vi "Process.CreateRefs.vi"(7 "Default IDs":u32[](array[numeric]), 8 "error in (no error)":errorcluster, 10 "Port Settings":T1, 11 "Name":string) -> (0 "error out":errorcluster, 2 "FilterDVR.Ref":refnum<data-value>, 3 "Initial Settings":T5)   [LabVIEW 2025, in "xnet_can_bus_monitor_api_server_do.lvlib"]
uses:
  Types/XNET.InitialSettings.ctl
  xnet_can_bus_monitor_api_server/RPC Messages/ni_xnet_can_bm_api_ConnectSettings.ctl
  xnet_can_bus_monitor_api_server/RPC Messages/ni_xnet_can_bm_api_CanMode.ctl
  xnet_can_bus_monitor_api_server/RPC Messages/ni_xnet_can_bm_api_Termination.ctl
  xnet_can_bus_monitor_api_server/RPC Messages/ni_xnet_can_bm_api_FdIsoMode.ctl
  xnet_can_bus_monitor_api_server/RPC Messages/ni_xnet_can_bm_api_FilterInfo.ctl
  xnet_can_bus_monitor_api_server/RPC Messages/ni_xnet_can_bm_api_DirectionFilter.ctl
  xnet_can_bus_monitor_api_server/RPC Messages/ni_xnet_can_bm_api_FrameFilter.ctl
  xnet_can_bus_monitor_api_server_do.lvlib
  xnet_can_bus_monitor_api_server/xnet_can_bus_monitor_api_server.lvlib
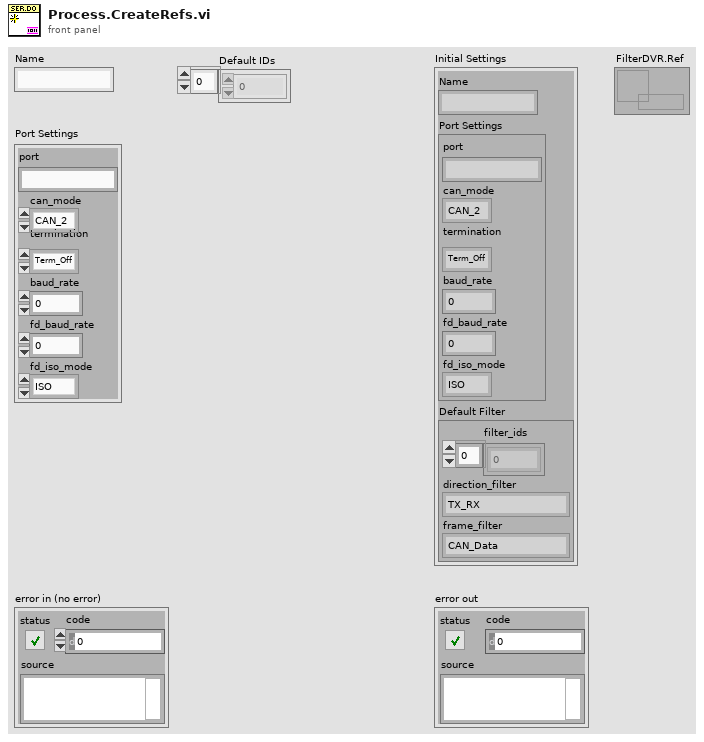
[diagram p1: front panel]
types:
  T1 = typedef "xnet_can_bus_monitor_api_server.lvlib/ni_xnet_can_bm_api_ConnectSettings.ctl" = cluster{"port":string, "can_mode":T2, "termination":T3, "baud_rate":u64, "fd_baud_rate":u64, "fd_iso_mode":T4}
  T2 = typedef "xnet_can_bus_monitor_api_server.lvlib/ni_xnet_can_bm_api_CanMode.ctl" = enum32{"CAN_2", "CAN_FD", "CAN_FD_BRS"}
  T3 = typedef "xnet_can_bus_monitor_api_server.lvlib/ni_xnet_can_bm_api_Termination.ctl" = enum32{"Term_Off", "Term_On"}
  T4 = typedef "xnet_can_bus_monitor_api_server.lvlib/ni_xnet_can_bm_api_FdIsoMode.ctl" = enum32{"ISO", "Non_ISO", "ISO_Legacy"}
  T5 = typedef "xnet_can_bus_monitor_api_server_do.lvlib/XNET.InitialSettings.ctl" = cluster{"Name":string, "Port Settings":T1, "Default Filter":T6}
  T6 = typedef "xnet_can_bus_monitor_api_server.lvlib/ni_xnet_can_bm_api_FilterInfo.ctl" = cluster{"filter_ids":u32[], "direction_filter":T7, "frame_filter":T8}
  T7 = typedef "xnet_can_bus_monitor_api_server.lvlib/ni_xnet_can_bm_api_DirectionFilter.ctl" = enum32{"TX_RX", "RX", "TX"}
  T8 = typedef "xnet_can_bus_monitor_api_server.lvlib/ni_xnet_can_bm_api_FrameFilter.ctl" = enum32{"CAN_Data", "CAN_Remote", "CAN_Bus_Error", "CAN_2_Data", "CAN_FD_Data", "CAN_FD_BRS_Data", "J1939_Data", "Delay", "Log_Trigger", "Start_Trigger", "All"}
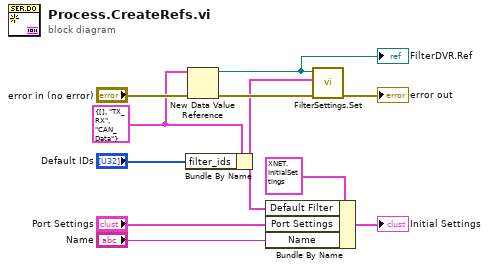
[diagram p0: block diagram]
diagram:
  w4 = T6 {"filter_ids"=[], "direction_filter"=enum."TX_RX", "frame_filter"=enum."CAN_Data"} ("Default Filter")
  n1 = Bundle By Name(cluster=w4, "filter_ids"="Default IDs") -> (w1:T6)
  n2 = New Data Value Reference(data value=w4, error in="error in (no error)") -> (data value reference=w2:refnum<data-value>, error out=w7:errorcluster)
  "FilterDVR.Ref" <- w2
  n3 = Bundle By Name(cluster=T5 {"Name"="", "Port Settings"={"port"="", "can_mode"=enum."CAN_2", "termination"=enum."Term_Off", "baud_rate"=0, "fd_baud_rate"=0, "fd_iso_mode"=enum."ISO"}, "Default Filter"={"filter_ids"=[], "direction_filter"=enum."TX_RX", "frame_filter"=enum."CAN_Data"}}, "Default Filter"=w1, "Port Settings"="Port Settings", "Name"="Name") -> (→"Initial Settings":T5)
  n4 = call "FilterSettings.Set.vi"("error in (no error)"=w7, "Filter"=w1, "FilterDVR.Ref"=w2) -> ("error out"=→"error out":errorcluster)  [unwired: 8 in]
